vi "SENS_SEGM_X_SPAC.vi"(0 "VISA IN":refnum<visa-resource-name>, 1 "Segment":i32=1, 2 "X-Axis Point Spacing(LINear or OBASe)":string(combo)="LINear", 5 "error in":errorcluster, 7 "Channel":i32=1) -> (14 "VISA Out":refnum<visa-resource-name>, 19 "error out":errorcluster)   [LabVIEW 2018, in "PNA-X.lvlib"]
doc: "SENSe<cnum>:SEGMent<snum>:X:SPACing <char> \n(Read-Write) Sets X-axis spacing ON or OFF \nParameters \n<cnum> Any existing channel number. If unspecified, value is set to 1 \n<snum> Any existing segment number. (This parameter is ignored) \n<char> LINear - turns X-axis point spacing OFF \nOBASe - turns X-axis point spacing ON \nExamples SENS:SEGM:X:SPACing LIN \nsense2:segment1:spacing obase \nQuery Syntax SENSe<cnum>:SEGMent<snum>:X:SPACing? \nReturn Type Character \nDefault LINear \n1814\n\nSense:Sweep Commands \nSpecifies the sweep functions of the analyzer. \nClick on a blue keyword to view the command details. \nSee Also \nExample Programs \nExample Triggering the PNA using SCPI \nLearn about Sweeping \nSynchronizing the PNA and Controller \nSCPI Command Tree \nNote: All of the commands in this block will accept MIN or MAX instead of a numeric parameter. \nAlso, kHZ, MHz, and GHz are accepted as suffixes/units. \nSee SCPI Syntax for more information."
uses:
  PNA-X.lvlib
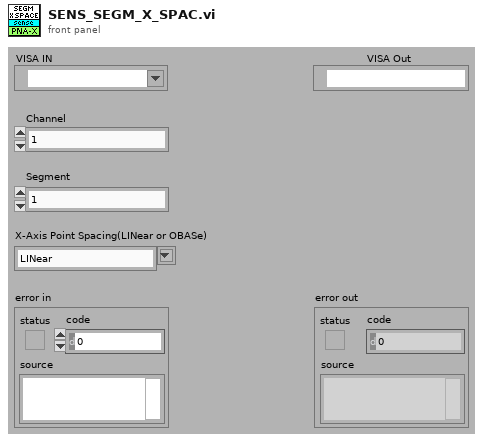
[diagram p1: front panel]
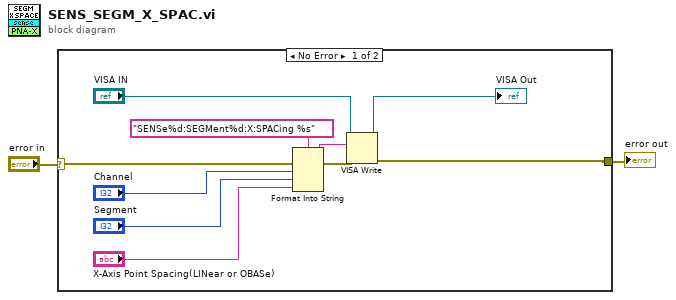
[diagram p0: block diagram]
diagram:
  n1 = case shown="No Error" "error in" {
    selector: "error in" -> [w12 w13]
    tunnel: [w7 w13] -> w1
    frame No Error {
      n2 = Format Into String(format string="SENSe%d:SEGMent%d:X:SPACing %s" ("Cmdline"), error in=w12, "Channel", "Segment", "X-Axis Point Spacing(LINear or OBASe)") -> (resulting string=w10:string, error out=w11:errorcluster)  [unwired: 1 in]
      n3 = VISA Write(VISA resource name="VISA IN", write buffer=w10, error in (no error)=w11) -> (VISA resource name out=→"VISA Out":refnum<visa-resource-name>, error out=w7:errorcluster)  [unwired: 1 out]
    }
    frame Error {
    }
  }
  "error out" <- w1
